vi "Read HalfVSS.vi"(8 "error in (no error)":errorcluster, 11 "Referee in":refnum<class "Referee.lvclass">) -> (0 "error out":errorcluster, 2 "HalfVSS":enum16{"SECOND_HALF", "FIRST_HALF", "NO_HALF"}(ring), 3 "Referee out":refnum<class "Referee.lvclass">)   [LabVIEW 2020, in "Referee.lvclass"]
uses:
  Referee.lvclass
  Referee.lvclass/Referee.ctl
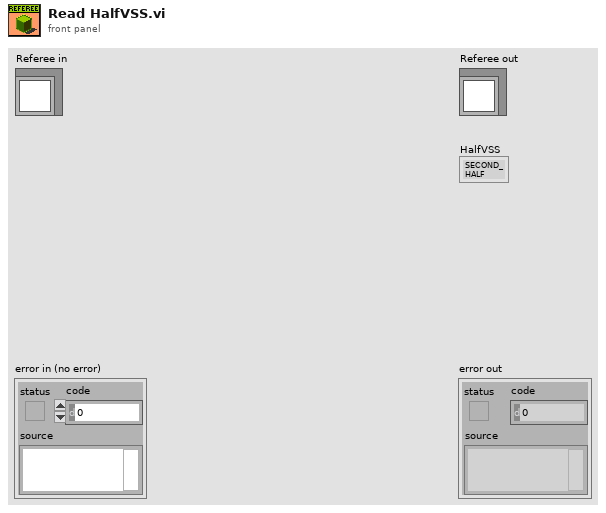
[diagram p1: front panel]
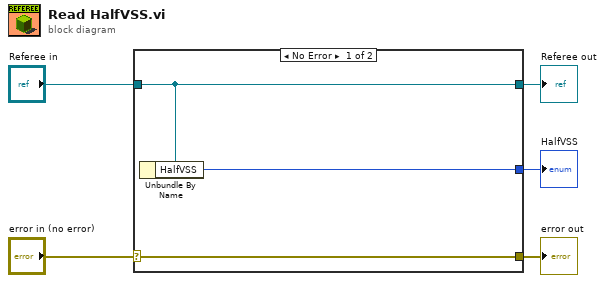
[diagram p0: block diagram]
diagram:
  n1 = case shown="No Error" "error in (no error)" {
    selector: "error in (no error)" -> [w8 w9]
    tunnel: [w8 w9] -> w4
    tunnel: [w7 w10] -> w2
    tunnel: "Referee in" -> [w7 w10]
    tunnel: [w6 _] -> w1
    frame No Error {
      n2 = Unbundle By Name(w7) -> ("HalfVSS"=w6:enum16{"SECOND_HALF", "FIRST_HALF", "NO_HALF"})
    }
    frame Error {
    }
  }
  "error out" <- w4
  "Referee out" <- w2
  "HalfVSS" <- w1
